vi "My Golden Section 1D.vi"(1 "Array In":dbl[](array[numeric])=[7.044400000000002, 0.4286399999999992, 0.536279999999991, 1.5500139999999916, 0.17059000000000035, 0.35147, 0.30979, 0.04216999999999992, 7.418052057077897] format="%_4g", 2 "d":dbl=1e-05 format="%_4g", 3 "# Points":i32=15, 4 "Var":u32=7) -> (0 "Array Out":dbl[](array[numeric])=[7.044400000000002, 0.4286399999999992, 0.536279999999991, 1.5500139999999916, 0.17059000000000035, 0.35147, 0.30979, 0.04216999999999992, 7.418052057077897] format="%_4g")   [LabVIEW 2016]
panel:
  in  "Iterate?":bool=TRUE
  out "XY Graph":cluster{dbl[], dbl[]}(graph)={[0.04202999999999992, 0.042039999999999925, 0.04204999999999992, 0.042059999999999924, 0.04206999999999992, 0.04207999999999992, 0.042089999999999926, 0.04209999999999992, 0.042109999999999925, 0.04211999999999992, 0.042129999999999924, 0.04213999999999992, 0.042149999999999924, 0.04215999999999992, 0.04216999999999992, 0.04216999999999992, 0.042179999999999926, 0.04218999999999992, 0.042199999999999925, 0.04220999999999992, 0.042219999999999924, 0.04222999999999992, 0.04223999999999992, 0.04224999999999992, 0.04225999999999992, 0.042269999999999926, 0.04227999999999992, 0.042289999999999925, 0.04229999999999992, 0.042309999999999924], [7.428454944255646, 7.426979859429947, 7.42561761370846, 7.424368151935538, 7.423231418974126, 7.422207359705648, 7.421295919030079, 7.4204970418659375, 7.4198106731502245, 7.419236757838441, 7.418775240904679, 7.418426067341454, 7.418189182159813, 7.418064530389271, 7.418052057077897, 7.418052057077897, 7.418151707292125, 7.418363426116984, 7.418687158655915, 7.419122850030831, 7.419670445382129, 7.420329889868631, 7.421101128667647, 7.421984106974895, 7.422978770004574, 7.424085062989279, 7.425302931180083, 7.426632319846432, 7.428073174276247, 7.4296254397758155]}
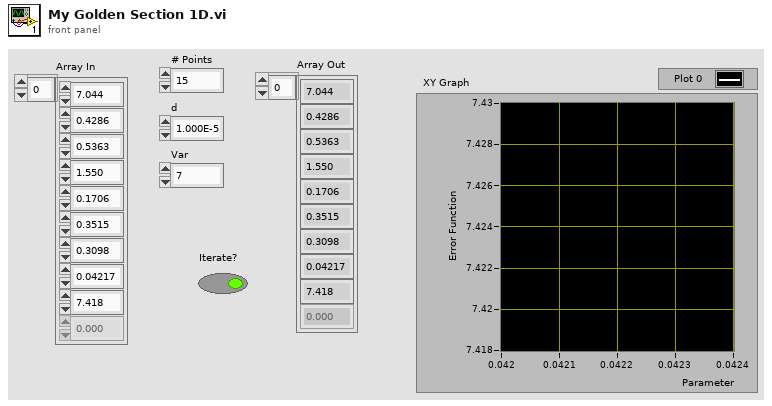
[diagram p1: front panel]
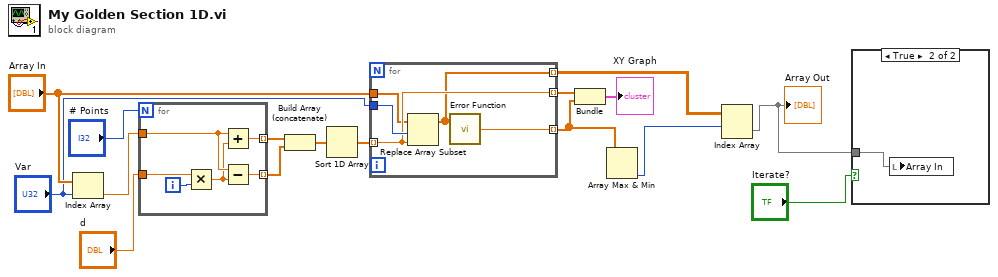
[diagram p0: block diagram]
diagram:
  n1 = Index Array(array="Array In", index="Var") -> (element=w15:dbl)
  n2 = for {
    N: "# Points" -> [_]
    tunnel: w15 -> [w19]
    tunnel: "d" -> [w22]
    tunnel: [w20] -> w7 mode=indexing
    tunnel: [w17] -> w8 mode=indexing
    i -> [w21]
    n3 = Multiply(x=w22, y=w21) -> (x*y=w18:dbl)
    n4 = Add(x=w19, y=w18) -> (x+y=w20:dbl)
    n5 = Subtract(x=w19, y=w18) -> (x-y=w17:dbl)
  }
  n6 = Build Array (concatenate)(w7, w8) -> (w6:dbl[])
  n7 = Sort 1D Array(array=w6) -> (sorted array=w13:dbl[])
  n8 = for {
    tunnel: w13 -> [w25] mode=indexing
    tunnel: "Array In" -> [w24]
    tunnel: "Var" -> [w27]
    tunnel: [w26] -> w5 mode=indexing
    tunnel: [w25] -> w9 mode=indexing
    tunnel: [w23] -> w4 mode=indexing
    n9 = Replace Array Subset(array=w24, new element=w25, index=w27) -> (w23:dbl[])
    n10 = call "Error Function.vi"("Array"=w23) -> ("Error"=w26:dbl)  [unwired: 1 in]
  }
  n11 = Bundle(w9, w5) -> (→"XY Graph":cluster{dbl[], dbl[]})  [unwired: 1 in]
  n12 = Array Max & Min(array=w5) -> (min index (indices)=w3:i32)  [unwired: 3 out]
  n13 = Index Array(array=w4, index (row)=w3) -> (element=w2:dbl[])  [unwired: 1 in]
  "Array Out" <- w2
  n14 = case shown="True" "Iterate?" {
    tunnel: w2 -> [_ w28]
    frame False {
    }
    frame True {
      n15 = local write "Array In"(w28) -> ()
    }
  }
